vi "Methods_Insert Dividers.vi"(11 "Methods[] In":T1(array[cluster])) -> (3 "Methods[] Out":T1(array[cluster]))   [LabVIEW 2023] (continued)
"Short name (localized)"="ClearSpecCompObjCache", "Long name (localized)"="Clear Specific Compiled Object Cache"}, "Method Flags"={"IsDeprecated"=FALSE, "IsPrivate"=TRUE, "IsScripting"=FALSE, "IsNotInRun-Time"=TRUE}, "Divider"=FALSE}, {"Class Info"={"Unique ID string"="1", "Parent ID string"="", "Class Name (unlocalized)"="Application", "Class Name (localized)"="Application"}, "Method Info"={"Unique ID string"="969", "Data name"="Restart", "Short name (localized)"="Restart", "Long name (localized)"="Restart"}, "Method Flags"={"IsDeprecated"=FALSE, "IsPrivate"=FALSE, "IsScripting"=FALSE, "IsNotInRun-Time"=FALSE}, "Divider"=FALSE}, {"Class Info"={"Unique ID string"="1", "Parent ID string"="", "Class Name (unlocalized)"="Application", "Class Name (localized)"="Application"}, "Method Info"={"Unique ID string"="970", "Data name"="Get Compiled Object File", "Short name (localized)"="Get Compiled Object File", "Long name (localized)"="GetCompiledObjectFile"}, "Method Flags"={"IsDeprecated"=FALSE, "IsPrivate"=TRUE, "IsScripting"=FALSE, "IsNotInRun-Time"=FALSE}, "Divider"=FALSE}, {"Class Info"={"Unique ID string"="1", "Parent ID string"="", "Class Name (unlocalized)"="Application", "Class Name (localized)"="Application"}, "Method Info"={"Unique ID string"="971", "Data name"="ClearAppBuilderCache", "Short name (localized)"="ClearAppBuilderCache", "Long name (localized)"="Clear Application Builder Cache"}, "Method Flags"={"IsDeprecated"=FALSE, "IsPrivate"=FALSE, "IsScripting"=FALSE, "IsNotInRun-Time"=TRUE}, "Divider"=FALSE}, {"Class Info"={"Unique ID string"="1", "Parent ID string"="", "Class Name (unlocalized)"="Application", "Class Name (localized)"="Application"}, "Method Info"={"Unique ID string"="972", "Data name"="TracingTimerEnable", "Short name (localized)"="TracingTimerEnable", "Long name (localized)"="Tracing Timer Enable"}, "Method Flags"={"IsDeprecated"=FALSE, "IsPrivate"=TRUE, "IsScripting"=FALSE, "IsNotInRun-Time"=TRUE}, "Divider"=FALSE}, {"Class Info"={"Unique ID string"="1", "Parent ID string"="", "Class Name (unlocalized)"="Application", "Class Name (localized)"="Application"}, "Method Info"={"Unique ID string"="973", "Data name"="TracingTimerHarvestLogAndReset", "Short name (localized)"="TracingTimerHarvestLogAndReset", "Long name (localized)"="Tracing Timer Harvest Log And Reset"}, "Method Flags"={"IsDeprecated"=FALSE, "IsPrivate"=TRUE, "IsScripting"=FALSE, "IsNotInRun-Time"=TRUE}, "Divider"=FALSE}, {"Class Info"={"Unique ID string"="1", "Parent ID string"="", "Class Name (unlocalized)"="Application", "Class Name (localized)"="Application"}, "Method Info"={"Unique ID string"="974", "Data name"="Context.CrossContextLoadVI", "Short name (localized)"="Context.CrossContextLoadVI", "Long name (localized)"="Context:Cross Context Load Unsaved VI"}, "Method Flags"={"IsDeprecated"=FALSE, "IsPrivate"=TRUE, "IsScripting"=FALSE, "IsNotInRun-Time"=FALSE}, "Divider"=FALSE}, {"Class Info"={"Unique ID string"="1", "Parent ID string"="", "Class Name (unlocalized)"="Application", "Class Name (localized)"="Application"}, "Method Info"={"Unique ID string"="978", "Data name"="Freeze Polys", "Short name (localized)"="Freeze Polys", "Long name (localized)"="Freeze Poly VIs"}, "Method Flags"={"IsDeprecated"=FALSE, "IsPrivate"=TRUE, "IsScripting"=FALSE, "IsNotInRun-Time"=TRUE}, "Divider"=FALSE}, {"Class Info"={"Unique ID string"="1", "Parent ID string"="", "Class Name (unlocalized)"="Application", "Class Name (localized)"="Application"}, "Method Info"={"Unique ID string"="979", "Data name"="GetInstantiationVIPath", "Short name (localized)"="GetInstantiationVIPath", "Long name (localized)"="Get Instantiation VI Path"}, "Method Flags"={"IsDeprecated"=FALSE, "IsPrivate"=TRUE, "IsScripting"=FALSE, "IsNotInRun-Time"=FALSE}, "Divider"=FALSE}, {"Class Info"={"Unique ID string"="1", "Parent ID string"="", "Class Name (unlocalized)"="Application", "Class Name (localized)"="Application"}, "Method Info"={"Unique ID string"="97a", "Data name"="Change Popup Paths", "Short name (localized)"="Change Popup Paths", "Long name (localized)"="Change Control Popup RTM Paths"}, "Method Flags"={"IsDeprecated"=FALSE, "IsPrivate"=TRUE, "IsScripting"=FALSE, "IsNotInRun-Time"=TRUE}, "Divider"=FALSE}, {"Class Info"={"Unique ID string"="1", "Parent ID string"="", "Class Name (unlocalized)"="Application", "Class Name (localized)"="Application"}, "Method Info"={"Unique ID string"="97b", "Data name"="Project.NewWithPrompts", "Short name (localized)"="Project.NewWithPrompts", "Long name (localized)"="Project:New with Prompts"}, "Method Flags"={"IsDeprecated"=FALSE, "IsPrivate"=FALSE, "IsScripting"=TRUE, "IsNotInRun-Time"=TRUE}, "Divider"=FALSE}, {"Class Info"={"Unique ID string"="1", "Parent ID string"="", "Class Name (unlocalized)"="Application", "Class Name (localized)"="Application"}, "Method Info"={"Unique ID string"="97c", "Data name"="ResetCrossCompileCount", "Short name (localized)"="ResetCrossCompileCount", "Long name (localized)"="Reset Cross Compile Count"}, "Method Flags"={"IsDeprecated"=FALSE, "IsPrivate"=TRUE, "IsScripting"=FALSE, "IsNotInRun-Time"=TRUE}, "Divider"=FALSE}, {"Class Info"={"Unique ID string"="1", "Parent ID string"="", "Class Name (unlocalized)"="Application", "Class Name (localized)"="Application"}, "Method Info"={"Unique ID string"="97d", "Data name"="Get Broken VI List", "Short name (localized)"="Get Broken VI List", "Long name (localized)"="Get Broken VI List"}, "Method Flags"={"IsDeprecated"=FALSE, "IsPrivate"=TRUE, "IsScripting"=TRUE, "IsNotInRun-Time"=TRUE}, "Divider"=FALSE}, {"Class Info"={"Unique ID string"="1", "Parent ID string"="", "Class Name (unlocalized)"="Application", "Class Name (localized)"="Application"}, "Method Info"={"Unique ID string"="97e", "Data name"="Get VI.Is Global", "Short name (localized)"="Get VI.Is Global", "Long name (localized)"="Get VI:Is Global"}, "Method Flags"={"IsDeprecated"=FALSE, "IsPrivate"=TRUE, "IsScripting"=FALSE, "IsNotInRun-Time"=TRUE}, "Divider"=FALSE}, {"Class Info"={"Unique ID string"="1", "Parent ID string"="", "Class Name (unlocalized)"="Application", "Class Name (localized)"="Application"}, "Method Info"={"Unique ID string"="97f", "Data name"="Get VI.CompiledForCurrent", "Short name (localized)"="Get VI.CompiledForCurrent", "Long name (localized)"="Get VI:Compiled For Current"}, "Method Flags"={"IsDeprecated"=FALSE, "IsPrivate"=TRUE, "IsScripting"=FALSE, "IsNotInRun-Time"=TRUE}, "Divider"=FALSE}, {"Class Info"={"Unique ID string"="1", "Parent ID string"="", "Class Name (unlocalized)"="Application", "Class Name (localized)"="Application"}, "Method Info"={"Unique ID string"="980", "Data name"="LoadMSCompilerComponent", "Short name (localized)"="LoadMSCompilerComponent", "Long name (localized)"="MathScript:Load MathScript Compiler Component"}, "Method Flags"={"IsDeprecated"=FALSE, "IsPrivate"=TRUE, "IsScripting"=FALSE, "IsNotInRun-Time"=TRUE}, "Divider"=FALSE}, {"Class Info"={"Unique ID string"="1", "Parent ID string"="", "Class Name (unlocalized)"="Application", "Class Name (localized)"="Application"}, "Method Info"={"Unique ID string"="981", "Data name"="Refresh Menus", "Short name (localized)"="Refresh Menus", "Long name (localized)"="Menus:Refresh"}, "Method Flags"={"IsDeprecated"=FALSE, "IsPrivate"=FALSE, "IsScripting"=FALSE, "IsNotInRun-Time"=TRUE}, "Divider"=FALSE}, {"Class Info"={"Unique ID string"="1", "Parent ID string"="", "Class Name (unlocalized)"="Application", "Class Name (localized)"="Application"}, "Method Info"={"Unique ID string"="982", "Data name"="Library.Has Shared Variables", "Short name (localized)"="Library.Has Shared Variables", "Long name (localized)"="Library:Has Shared Variables"}, "Method Flags"={"IsDeprecated"=FALSE, "IsPrivate"=TRUE, "IsScripting"=FALSE, "IsNotInRun-Time"=TRUE}, "Divider"=FALSE}, {"Class Info"={"Unique ID string"="1", "Parent ID string"="", "Class Name (unlocalized)"="Application", "Class Name (localized)"="Application"}, "Method Info"={"Unique ID string"="983", "Data name"="UI.Cmp VIs XML", "Short name (localized)"="UI.Cmp VIs XML", "Long name (localized)"="User Interaction:Compare VIs XML"}, "Method Flags"={"IsDeprecated"=FALSE, "IsPrivate"=TRUE, "IsScripting"=FALSE, "IsNotInRun-Time"=TRUE}, "Divider"=FALSE}, {"Class Info"={"Unique ID string"="1", "Parent ID string"="", "Class Name (unlocalized)"="Application", "Class Name (localized)"="Application"}, "Method Info"={"Unique ID string"="985", "Data name"="Object Manager:Get Managers", "Short name (localized)"="Object Manager:Get Managers", "Long name (localized)"="Object Manager:Get Managers"}, "Method Flags"={"IsDeprecated"=FALSE, "IsPrivate"=TRUE, "IsScripting"=FALSE, "IsNotInRun-Time"=FALSE}, "Divider"=FALSE}, {"Class Info"={"Unique ID string"="1", "Parent ID string"="", "Class Name (unlocalized)"="Application", "Class Name (localized)"="Application"}, "Method Info"={"Unique ID string"="986", "Data name"="Object Manager:Get Classes", "Short name (localized)"="Object Manager:Get Classes", "Long name (localized)"="Object Manager:Get Classes"}, "Method Flags"={"IsDeprecated"=FALSE, "IsPrivate"=TRUE, "IsScripting"=FALSE, "IsNotInRun-Time"=FALSE}, "Divider"=FALSE}, {"Class Info"={"Unique ID string"="1", "Parent ID string"="", "Class Name (unlocalized)"="Application", "Class Name (localized)"="Application"}, "Method Info"={"Unique ID string"="987", "Data name"="Object Manager:Get Properties", "Short name (localized)"="Object Manager:Get Properties", "Long name (localized)"="Object Manager:Get Properties"}, "Method Flags"={"IsDeprecated"=FALSE, "IsPrivate"=TRUE, "IsScripting"=FALSE, "IsNotInRun-Time"=FALSE}, "Divider"=FALSE}, {"Class Info"={"Unique ID string"="1", "Parent ID string"="", "Class Name (unlocalized)"="Application", "Class Name (localized)"="Application"}, "Method Info"={"Unique ID string"="988", "Data name"="Object Manager:Show Help", "Short name (localized)"="Object Manager:Show Help", "Long name (localized)"="Object Manager:Show Help"}, "Method Flags"={"IsDeprecated"=FALSE, "IsPrivate"=TRUE, "IsScripting"=FALSE, "IsNotInRun-Time"=FALSE}, "Divider"=FALSE}, {"Class Info"={"Unique ID string"="1", "Parent ID string"="", "Class Name (unlocalized)"="Application", "Class Name (localized)"="Application"}, "Method Info"={"Unique ID string"="989", "Data name"="Get VI.Bookmarks", "Short name (localized)"="Get VI.Bookmarks", "Long name (localized)"="Get VI:Bookmarks"}, "Method Flags"={"IsDeprecated"=FALSE, "IsPrivate"=FALSE, "IsScripting"=FALSE, "IsNotInRun-Time"=FALSE}, "Divider"=FALSE}, {"Class Info"={"Unique ID string"="1", "Parent ID string"="", "Class Name (unlocalized)"="Application", "Class Name (localized)"="Application"}, "Method Info"={"Unique ID string"="98a", "Data name"="DoPostInstallObjCacheCheck", "Short name (localized)"="DoPostInstallObjCacheCheck", "Long name (localized)"="Do Post Install ObjCache Check"}, "Method Flags"={"IsDeprecated"=FALSE, "IsPrivate"=TRUE, "IsScripting"=FALSE, "IsNotInRun-Time"=TRUE}, "Divider"=FALSE}, {"Class Info"={"Unique ID string"="1", "Parent ID string"="", "Class Name (unlocalized)"="Application", "Class Name (localized)"="Application"}, "Method Info"={"Unique ID string"="98b", "Data name"="All Methods Of LVClass", "Short name (localized)"="All Methods Of LVClass", "Long name (localized)"="LabVIEW Class:All Methods of LVClass"}, "Method Flags"={"IsDeprecated"=FALSE, "IsPrivate"=FALSE, "IsScripting"=FALSE, "IsNotInRun-Time"=FALSE}, "Divider"=FALSE}, {"Class Info"={"Unique ID string"="1", "Parent ID string"="", "Class Name (unlocalized)"="Application", "Class Name (localized)"="Application"}, "Method Info"={"Unique ID string"="98c", "Data name"="LVClass Implementing VI Path", "Short name (localized)"="LVClass Implementing VI Path", "Long name (localized)"="LabVIEW Class:Get Implementing VI Path"}, "Method Flags"={"IsDeprecated"=FALSE, "IsPrivate"=FALSE, "IsScripting"=FALSE, "IsNotInRun-Time"=FALSE}, "Divider"=FALSE}, {"Class Info"={"Unique ID string"="1", "Parent ID string"="", "Class Name (unlocalized)"="Application", "Class Name (localized)"="Application"}, "Method Info"={"Unique ID string"="98d", "Data name"="Get VI.GetPrimDeps", "Short name (localized)"="Get VI.GetPrimDeps", "Long name (localized)"="Get VI:Get Prim Dependency Flags"}, "Method Flags"={"IsDeprecated"=FALSE, "IsPrivate"=TRUE, "IsScripting"=TRUE, "IsNotInRun-Time"=TRUE}, "Divider"=FALSE}, {"Class Info"={"Unique ID string"="1", "Parent ID string"="", "Class Name (unlocalized)"="Application", "Class Name (localized)"="Application"}, "Method Info"={"Unique ID string"="98e", "Data name"="IsCalleeInlined", "Short name (localized)"="IsCalleeInlined", "Long name (localized)"="Compiler:Is Callee Inlined"}, "Method Flags"={"IsDeprecated"=FALSE, "IsPrivate"=TRUE, "IsScripting"=FALSE, "IsNotInRun-Time"=FALSE}, "Divider"=FALSE}, {"Class Info"={"Unique ID string"="1", "Parent ID string"="", "Class Name (unlocalized)"="Application", "Class Name (localized)"="Application"}, "Method Info"={"Unique ID string"="98f", "Data name"="UI.ShowPaletteObjContextHelp", "Short name (localized)"="UI.ShowPaletteObjContextHelp", "Long name (localized)"="User Interaction:Show Palette Object Context Help"}, "Method Flags"={"IsDeprecated"=FALSE, "IsPrivate"=FALSE, "IsScripting"=TRUE, "IsNotInRun-Time"=TRUE}, "Divider"=FALSE}, {"Class Info"={"Unique ID string"="1", "Parent ID string"="", "Class Name (unlocalized)"="Application", "Class Name (localized)"="Application"}, "Method Info"={"Unique ID string"="990", "Data name"="Get VI.Help Info", "Short name (localized)"="Get VI.Help Info", "Long name (localized)"="Get VI:Help Info"}, "Method Flags"={"IsDeprecated"=FALSE, "IsPrivate"=FALSE, "IsScripting"=FALSE, "IsNotInRun-Time"=FALSE}, "Divider"=FALSE}, {"Class Info"={"Unique ID string"="1", "Parent ID string"="", "Class Name (unlocalized)"="Application", "Class Name (localized)"="Application"}, "Method Info"={"Unique ID string"="991", "Data name"="DSObserverCmd", "Short name (localized)"="DSObserverCmd", "Long name (localized)"="Memory Profiling:DSObserver Command"}, "Method Flags"={"IsDeprecated"=FALSE, "IsPrivate"=TRUE, "IsScripting"=FALSE, "IsNotInRun-Time"=FALSE}, "Divider"=FALSE}, {"Class Info"={"Unique ID string"="1", "Parent ID string"="", "Class Name (unlocalized)"="Application", "Class Name (localized)"="Application"}, "Method Info"={"Unique ID string"="992", "Data name"="OpenBinaryLibrary", "Short name (localized)"="OpenBinaryLibrary", "Long name (localized)"="OpenBinaryLibrary"}, "Method Flags"={"IsDeprecated"=FALSE, "IsPrivate"=TRUE, "IsScripting"=FALSE, "IsNotInRun-Time"=FALSE}, "Divider"=FALSE}, {"Class Info"={"Unique ID string"="1", "Parent ID string"="", "Class Name (unlocalized)"="Application", "Class Name (localized)"="Application"}, "Method Info"={"Unique ID string"="993", "Data name"="CloseLEIFBuildData", "Short name (localized)"="CloseLEIFBuildData", "Long name (localized)"="Close LEIF Build Data Cookie"}, "Method Flags"={"IsDeprecated"=FALSE, "IsPrivate"=TRUE, "IsScripting"=FALSE, "IsNotInRun-Time"=TRUE}, "Divider"=FALSE}, {"Class Info"={"Unique ID string"="1", "Parent ID string"="", "Class Name (unlocalized)"="Application", "Class Name (localized)"="Application"}, "Method Info"={"Unique ID string"="994", "Data name"="Build.BCRTEEnabledPackedLibrary", "Short name (localized)"="Build.BCRTEEnabledPackedLibrary", "Long name (localized)"="Build:BCRTEEnabledPackedLibrary"}, "Method Flags"={"IsDeprecated"=FALSE, "IsPrivate"=TRUE, "IsScripting"=FALSE, "IsNotInRun-Time"=TRUE}, "Divider"=FALSE}, {"Class Info"={"Unique ID string"="1", "Parent ID string"="", "Class Name (unlocalized)"="Application", "Class Name (localized)"="Application"}, "Method Info"={"Unique ID string"="995", "Data name"="PackedLibrary.IsLoadableInBinaryCompatibleLV", "Short name (localized)"="PackedLibrary.IsLoadableInBinaryCompatibleLV", "Long name (localized)"="Packed Library:Is Packed Library Loadable In Binary Compatible LabVIEW"}, "Method Flags"={"IsDeprecated"=FALSE, "IsPrivate"=TRUE, "IsScripting"=FALSE, "IsNotInRun-Time"=FALSE}, "Divider"=FALSE}, {"Class Info"={"Unique ID string"="1", "Parent ID string"="", "Class Name (unlocalized)"="Application", "Class Name (localized)"="Application"}, "Method Info"={"Unique ID string"="996", "Data name"="SetGlobalBackwardCompatibleLoadEnabled", "Short name (localized)"="SetGlobalBackwardCompatibleLoadEnabled", "Long name (localized)"="BCRTE:SetGlobalBackwardCompatibleLoadEnabled"}, "Method Flags"={"IsDeprecated"=FALSE, "IsPrivate"=TRUE, "IsScripting"=FALSE, "IsNotInRun-Time"=FALSE}, "Divider"=FALSE}, {"Class Info"={"Unique ID string"="1", "Parent ID string"="", "Class Name (unlocalized)"="Application", "Class Name (localized)"="Application"}, "Method Info"={"Unique ID string"="997", "Data name"="IsGlobalBackwardCompatibleLoadEnabled", "Short name (localized)"="IsGlobalBackwardCompatibleLoadEnabled", "Long name (localized)"="BCRTE:IsGlobalBackwardCompatibleLoadEnabled"}, "Method Flags"={"IsDeprecated"=FALSE, "IsPrivate"=TRUE, "IsScripting"=FALSE, "IsNotInRun-Time"=FALSE}, "Divider"=FALSE}, {"Class Info"={"Unique ID string"="1", "Parent ID string"="", "Class Name (unlocalized)"="Application", "Class Name (localized)"="Application"}, "Method Info"={"Unique ID string"="998", "Data name"="Linker.Read Info From File Exclude LVRT Shipped Libs", "Short name (localized)"="Linker.Read Info From File Exclude LVRT Shipped Libs", "Long name (localized)"="Linker:Read Info From File Exclude LVRT Shipped Libs"}, "Method Flags"={"IsDeprecated"=FALSE, "IsPrivate"=TRUE, "IsScripting"=FALSE, "IsNotInRun-Time"=TRUE}, "Divider"=FALSE}, {"Class Info"={"Unique ID string"="1", "Parent ID string"="", "Class Name (unlocalized)"="Application", "Class Name (localized)"="Application"}, "Method Info"={"Unique ID string"="999", "Data name"="Project.Open And Suppress Source-Only", "Short name (localized)"="Project.Open And Suppress Source-Only", "Long name (localized)"="Project:Open And Suppress Source-Only"}, "Method Flags"={"IsDeprecated"=FALSE, "IsPrivate"=FALSE, "IsScripting"=TRUE, "IsNotInRun-Time"=TRUE}, "Divider"=FALSE}, {"Class Info"={"Unique ID string"="1", "Parent ID string"="", "Class Name (unlocalized)"="Application", "Class Name (localized)"="Application"}, "Method Info"={"Unique ID string"="99a", "Data name"="NativeEventTracingSetup", "Short name (localized)"="NativeEventTracingSetup", "Long name (localized)"="NativeEventTracing:Setup"}, "Method Flags"={"IsDeprecated"=FALSE, "IsPrivate"=TRUE, "IsScripting"=FALSE, "IsNotInRun-Time"=FALSE}, "Divider"=FALSE}, {"Class Info"={"Unique ID string"="1", "Parent ID string"="", "Class Name (unlocalized)"="Application", "Class Name (localized)"="Application"}, "Method Info"={"Unique ID string"="99b", "Data name"="Get VI.ConPane CRC v3", "Short name (localized)"="Get VI.ConPane CRC v3", "Long name (localized)"="Get VI:ConPane CRC v3"}, "Method Flags"={"IsDeprecated"=FALSE, "IsPrivate"=TRUE, "IsScripting"=FALSE, "IsNotInRun-Time"=FALSE}, "Divider"=FALSE}, {"Class Info"={"Unique ID string"="1", "Parent ID string"="", "Class Name (unlocalized)"="Application", "Class Name (localized)"="Application"}, "Method Info"={"Unique ID string"="99c", "Data name"="Get VI.ConPane CRC Ignore DD v2", "Short name (localized)"="Get VI.ConPane CRC Ignore DD v2", "Long name (localized)"="Get VI:ConPane CRC Ignore Dynamic Dispatch v2"}, "Method Flags"={"IsDeprecated"=FALSE, "IsPrivate"=TRUE, "IsScripting"=FALSE, "IsNotInRun-Time"=FALSE}, "Divider"=FALSE}, {"Class Info"={"Unique ID string"="2", "Parent ID string"="", "Class Name (unlocalized)"="VI", "Class Name (localized)"="VI"}, "Method Info"={"Unique ID string"="3e8", "Data name"="VI Strings.Export", "Short name (localized)"="VI Strings.Export", "Long name (localized)"="VI Strings:Export"}, "Method Flags"={"IsDeprecated"=FALSE, "IsPrivate"=FALSE, "IsScripting"=FALSE, "IsNotInRun-Time"=TRUE}, "Divider"=FALSE}, {"Class Info"={"Unique ID string"="2", "Parent ID string"="", "Class Name (unlocalized)"="VI", "Class Name (localized)"="VI"}, "Method Info"={"Unique ID string"="3e9", "Data name"="VI Strings.Import", "Short name (localized)"="VI Strings.Import", "Long name (localized)"="VI Strings:Import"}, "Method Flags"={"IsDeprecated"=FALSE, "IsPrivate"=FALSE, "IsScripting"=FALSE, "IsNotInRun-Time"=FALSE}, "Divider"=FALSE}, {"Class Info"={"Unique ID string"="2", "Parent ID string"="", "Class Name (unlocalized)"="VI", "Class Name (localized)"="VI"}, "Method Info"={"Unique ID string"="3ea", "Data name"="Save.Instrument", "Short name (localized)"="Save.Instrument", "Long name (localized)"="Save:Instrument"}, "Method Flags"={"IsDeprecated"=FALSE, "IsPrivate"=FALSE, "IsScripting"=FALSE, "IsNotInRun-Time"=TRUE}, "Divider"=FALSE}, {"Class Info"={"Unique ID string"="2", "Parent ID string"="", "Class Name (unlocalized)"="VI", "Class Name (localized)"="VI"}, "Method Info"={"Unique ID string"="3eb", "Data name"="Run VI", "Short name (localized)"="Run VI", "Long name (localized)"="Run VI"}, "Method Flags"={"IsDeprecated"=FALSE, "IsPrivate"=FALSE, "IsScripting"=FALSE, "IsNotInRun-Time"=FALSE}, "Divider"=FALSE}, {"Class Info"={"Unique ID string"="2", "Parent ID string"="", "Class Name (unlocalized)"="VI", "Class Name (localized)"="VI"}, "Method Info"={"Unique ID string"="3ec", "Data name"="Abort VI", "Short name (localized)"="Abort VI", "Long name (localized)"="Abort VI"}, "Method Flags"={"IsDeprecated"=FALSE, "IsPrivate"=FALSE, "IsScripting"=FALSE, "IsNotInRun-Time"=FALSE}, "Divider"=FALSE}, {"Class Info"={"Unique ID string"="2", "Parent ID string"="", "Class Name (unlocalized)"="VI", "Class Name (localized)"="VI"}, "Method Info"={"Unique ID string"="3ed", "Data name"="Print.VI To Printer", "Short name (localized)"="Print.VI To Printer", "Long name (localized)"="Print:VI To Printer"}, "Method Flags"={"IsDeprecated"=FALSE, "IsPrivate"=FALSE, "IsScripting"=FALSE, "IsNotInRun-Time"=FALSE}, "Divider"=FALSE}, {"Class Info"={"Unique ID string"="2", "Parent ID string"="", "Class Name (unlocalized)"="VI", "Class Name (localized)"="VI"}, "Method Info"={"Unique ID string"="3ee", "Data name"="Print.VI To HTML", "Short name (localized)"="Print.VI To HTML", "Long name (localized)"="Print:VI To HTML"}, "Method Flags"={"IsDeprecated"=FALSE, "IsPrivate"=FALSE, "IsScripting"=FALSE, "IsNotInRun-Time"=TRUE}, "Divider"=FALSE}, {"Class Info"={"Unique ID string"="2", "Parent ID string"="", "Class Name (unlocalized)"="VI", "Class Name (localized)"="VI"}, "Method Info"={"Unique ID string"="3ef", "Data name"="Print.VI To RTF", "Short name (localized)"="Print.VI To RTF", "Long name (localized)"="Print:VI To RTF"}, "Method Flags"={"IsDeprecated"=FALSE, "IsPrivate"=FALSE, "IsScripting"=FALSE, "IsNotInRun-Time"=TRUE}, "Divider"=FALSE}, {"Class Info"={"Unique ID string"="2", "Parent ID string"="", "Class Name (unlocalized)"="VI", "Class Name (localized)"="VI"}, "Method Info"={"Unique ID string"="3f0", "Data name"="Print.VI To Text", "Short name (localized)"="Print.VI To Text", "Long name (localized)"="Print:VI To Text"}, "Method Flags"={"IsDeprecated"=FALSE, "IsPrivate"=FALSE, "IsScripting"=FALSE, "IsNotInRun-Time"=TRUE}, "Divider"=FALSE}, {"Class Info"={"Unique ID string"="2", "Parent ID string"="", "Class Name (unlocalized)"="VI", "Class Name (localized)"="VI"}, "Method Info"={"Unique ID string"="3f3", "Data name"="Default Vals.Make Curr Default", "Short name (localized)"="Default Vals.Make Curr Default", "Long name (localized)"="Default Values:Make Current Default"}, "Method Flags"={"IsDeprecated"=FALSE, "IsPrivate"=FALSE, "IsScripting"=FALSE, "IsNotInRun-Time"=TRUE}, "Divider"=FALSE}, {"Class Info"={"Unique ID string"="2", "Parent ID string"="", "Class Name (unlocalized)"="VI", "Class Name (localized)"="VI"}, "Method Info"={"Unique ID string"="3f4", "Data name"="Default Vals.Reinit All", "Short name (localized)"="Default Vals.Reinit All", "Long name (localized)"="Default Values:Reinitialize All To Default"}, "Method Flags"={"IsDeprecated"=FALSE, "IsPrivate"=FALSE, "IsScripting"=FALSE, "IsNotInRun-Time"=FALSE}, "Divider"=FALSE}, {"Class Info"={"Unique ID string"="2", "Parent ID string"="", "Class Name (unlocalized)"="VI", "Class Name (localized)"="VI"}, "Method Info"={"Unique ID string"="3fa", "Data name"="Revert VI", "Short name (localized)"="Revert VI", "Long name (localized)"="Revert VI"}, "Method Flags"={"IsDeprecated"=FALSE, "IsPrivate"=FALSE, "IsScripting"=FALSE, "IsNotInRun-Time"=TRUE}, "Divider"=FALSE}, {"Class Info"={"Unique ID string"="2", "Parent ID string"="", "Class Name (unlocalized)"="VI", "Class Name (localized)"="VI"}, "Method Info"={"Unique ID string"="3fb", "Data name"="Print.Panel To Printer", "Short name (localized)"="Print.Panel To Printer", "Long name (localized)"="Print:Panel To Printer"}, "Method Flags"={"IsDeprecated"=FALSE, "IsPrivate"=FALSE, "IsScripting"=FALSE, "IsNotInRun-Time"=FALSE}, "Divider"=FALSE}, {"Class Info"={"Unique ID string"="2", "Parent ID string"="", "Class Name (unlocalized)"="VI", "Class Name (localized)"="VI"}, "Method Info"={"Unique ID string"="3fd", "Data name"="Lock State.Get", "Short name (localized)"="Lock State.Get", "Long name (localized)"="Lock State:Get"}, "Method Flags"={"IsDeprecated"=FALSE, "IsPrivate"=FALSE, "IsScripting"=FALSE, "IsNotInRun-Time"=FALSE}, "Divider"=FALSE}, {"Class Info"={"Unique ID string"="2", "Parent ID string"="", "Class Name (unlocalized)"="VI", "Class Name (localized)"="VI"}, "Method Info"={"Unique ID string"="3fe", "Data name"="Lock State.Set", "Short name (localized)"="Lock State.Set", "Long name (localized)"="Lock State:Set"}, "Method Flags"={"IsDeprecated"=FALSE, "IsPrivate"=FALSE, "IsScripting"=FALSE, "IsNotInRun-Time"=TRUE}, "Divider"=FALSE}, {"Class Info"={"Unique ID string"="2", "Parent ID string"="", "Class Name (unlocalized)"="VI", "Class Name (localized)"="VI"}, "Method Info"={"Unique ID string"="3ff", "Data name"="Private Save Instrument", "Short name (localized)"="Private Save Instrument", "Long name (localized)"="Save:Instrument (Private)"}, "Method Flags"={"IsDeprecated"=FALSE, "IsPrivate"=TRUE, "IsScripting"=FALSE, "IsNotInRun-Time"=TRUE}, "Divider"=FALSE}, {"Class Info"={"Unique ID string"="2", "Parent ID string"="", "Class Name (unlocalized)"="VI", "Class Name (localized)"="VI"}, "Method Info"={"Unique ID string"="400", "Data name"="Save.For Previous", "Short name (localized)"="Save.For Previous", "Long name (localized)"="Save:For Previous"}, "Method Flags"={"IsDeprecated"=FALSE, "IsPrivate"=FALSE, "IsScripting"=FALSE, "IsNotInRun-Time"=TRUE}, "Divider"=FALSE}, {"Class Info"={"Unique ID string"="2", "Parent ID string"="", "Class Name (unlocalized)"="VI", "Class Name (localized)"="VI"}, "Method Info"={"Unique ID string"="401", "Data name"="Empty", "Short name (localized)"="Empty", "Long name (localized)"="Empty"}, "Method Flags"={"IsDeprecated"=FALSE, "IsPrivate"=FALSE, "IsScripting"=TRUE, "IsNotInRun-Time"=TRUE}, "Divider"=FALSE}, {"Class Info"={"Unique ID string"="2", "Parent ID string"="", "Class Name (unlocalized)"="VI", "Class Name (localized)"="VI"}, "Method Info"={"Unique ID string"="402", "Data name"="Transaction.Begin Undo", "Short name (localized)"="Transaction.Begin Undo", "Long name (localized)"="Transaction:Begin Undo"}, "Method Flags"={"IsDeprecated"=FALSE, "IsPrivate"=FALSE, "IsScripting"=TRUE, "IsNotInRun-Time"=TRUE}, "Divider"=FALSE}, {"Class Info"={"Unique ID string"="2", "Parent ID string"="", "Class Name (unlocalized)"="VI", "Class Name (localized)"="VI"}, "Method Info"={"Unique ID string"="403", "Data name"="Transaction.End Undo", "Short name (localized)"="Transaction.End Undo", "Long name (localized)"="Transaction:End Undo"}, "Method Flags"={"IsDeprecated"=FALSE, "IsPrivate"=FALSE, "IsScripting"=TRUE, "IsNotInRun-Time"=TRUE}, "Divider"=FALSE}, {"Class Info"={"Unique ID string"="2", "Parent ID string"="", "Class Name (unlocalized)"="VI", "Class Name (localized)"="VI"}, "Method Info"={"Unique ID string"="407", "Data name"="VI Icon.Set from File", "Short name (localized)"="VI Icon.Set from File", "Long name (localized)"="VI Icon:Set From File"}, "Method Flags"={"IsDeprecated"=FALSE, "IsPrivate"=FALSE, "IsScripting"=FALSE, "IsNotInRun-Time"=TRUE}, "Divider"=FALSE}, {"Class Info"={"Unique ID string"="2", "Parent ID string"="", "Class Name (unlocalized)"="VI", "Class Name (localized)"="VI"}, "Method Info"={"Unique ID string"="409", "Data name"="Tag.Remove Tags", "Short name (localized)"="Tag.Remove Tags", "Long name (localized)"="Tag:Remove Tags"}, "Method Flags"={"IsDeprecated"=FALSE, "IsPrivate"=TRUE, "IsScripting"=FALSE, "IsNotInRun-Time"=FALSE}, "Divider"=FALSE}, {"Class Info"={"Unique ID string"="2", "Parent ID string"="", "Class Name (unlocalized)"="VI", "Class Name (localized)"="VI"}, "Method Info"={"Unique ID string"="40a", "Data name"="Tag.Set Tags", "Short name (localized)"="Tag.Set Tags", "Long name (localized)"="Tag:Set Tags"}, "Method Flags"={"IsDeprecated"=FALSE, "IsPrivate"=TRUE, "IsScripting"=FALSE, "IsNotInRun-Time"=FALSE}, "Divider"=FALSE}, {"Class Info"={"Unique ID string"="2", "Parent ID string"="", "Class Name (unlocalized)"="VI", "Class Name (localized)"="VI"}, "Method Info"={"Unique ID string"="40b", "Data name"="Tag.Set Persistence", "Short name (localized)"="Tag.Set Persistence", "Long name (localized)"="Tag:Set Persistence"}, "Method Flags"={"IsDeprecated"=FALSE, "IsPrivate"=TRUE, "IsScripting"=FALSE, "IsNotInRun-Time"=FALSE}, "Divider"=FALSE}, {"Class Info"={"Unique ID string"="2", "Parent ID string"="", "Class Name (unlocalized)"="VI", "Class Name (localized)"="VI"}, "Method Info"={"Unique ID string"="40c", "Data name"="Tag.Remove All Tags", "Short name (localized)"="Tag.Remove All Tags", "Long name (localized)"="Tag:Remove All Tags"}, "Method Flags"={"IsDeprecated"=FALSE, "IsPrivate"=TRUE, "IsScripting"=FALSE, "IsNotInRun-Time"=FALSE}, "Divider"=FALSE}, {"Class Info"={"Unique ID string"="2", "Parent ID string"="", "Class Name (unlocalized)"="VI", "Class Name (localized)"="VI"}, "Method Info"={"Unique ID string"="40d", "Data name"="Tag.Set Tag", "Short name (localized)"="Tag.Set Tag", "Long name (localized)"="Tag:Set Tag"}, "Method Flags"={"IsDeprecated"=FALSE, "IsPrivate"=TRUE, "IsScripting"=FALSE, "IsNotInRun-Time"=FALSE}, "Divider"=FALSE}, {"Class Info"={"Unique ID string"="2", "Parent ID string"="", "Class Name (unlocalized)"="VI", "Class Name (localized)"="VI"}, "Method Info"={"Unique ID string"="40e", "Data name"="Tag.Get Tag", "Short name (localized)"="Tag.Get Tag", "Long name (localized)"="Tag:Get Tag"}, "Method Flags"={"IsDeprecated"=FALSE, "IsPrivate"=TRUE, "IsScripting"=FALSE, "IsNotInRun-Time"=FALSE}, "Divider"=FALSE}, {"Class Info"={"Unique ID string"="2", "Parent ID string"="", "Class Name (unlocalized)"="VI", "Class Name (localized)"="VI"}, "Method Info"={"Unique ID string"="40f", "Data name"="Tag.Remove Tag", "Short name (localized)"="Tag.Remove Tag", "Long name (localized)"="Tag:Remove Tag"}, "Method Flags"={"IsDeprecated"=FALSE, "IsPrivate"=TRUE, "IsScripting"=FALSE, "IsNotInRun-Time"=FALSE}, "Divider"=FALSE}, {"Class Info"={"Unique ID string"="2", "Parent ID string"="", "Class Name (unlocalized)"="VI", "Class Name (localized)"="VI"}, "Method Info"={"Unique ID string"="410", "Data name"="BD.Remove Bad Wires", "Short name (localized)"="BD.Remove Bad Wires", "Long name (localized)"="Block Diagram:Remove Bad Wires"}, "Method Flags"={"IsDeprecated"=FALSE, "IsPrivate"=FALSE, "IsScripting"=TRUE, "IsNotInRun-Time"=TRUE}, "Divider"=FALSE}, {"Class Info"={"Unique ID string"="2", "Parent ID string"="", "Class Name (unlocalized)"="VI", "Class Name (localized)"="VI"}, "Method Info"={"Unique ID string"="411", "Data name"="Fake Exec State", "Short name (localized)"="Fake Exec State", "Long name (localized)"="Fake Exec State"}, "Method Flags"={"IsDeprecated"=FALSE, "IsPrivate"=TRUE, "IsScripting"=TRUE, "IsNotInRun-Time"=FALSE}, "Divider"=FALSE}, {"Class Info"={"Unique ID string"="2", "Parent ID string"="", "Class Name (unlocalized)"="VI", "Class Name (localized)"="VI"}, "Method Info"={"Unique ID string"="412", "Data name"="Generate VHDL", "Short name (localized)"="Generate VHDL", "Long name (localized)"="Generate VHDL"}, "Method Flags"={"IsDeprecated"=FALSE, "IsPrivate"=TRUE, "IsScripting"=TRUE, "IsNotInRun-Time"=TRUE}, "Divider"=FALSE}, {"Class Info"={"Unique ID string"="2", "Parent ID string"="", "Class Name (unlocalized)"="VI", "Class Name (localized)"="VI"}, "Method Info"={"Unique ID string"="413", "Data name"="Save.Run-Time Menu", "Short name (localized)"="Save.Run-Time Menu", "Long name (localized)"="Save:Run-Time Menu"}, "Method Flags"={"IsDeprecated"=FALSE, "IsPrivate"=FALSE, "IsScripting"=FALSE, "IsNotInRun-Time"=TRUE}, "Divider"=FALSE}, {"Class Info"={"Unique ID string"="2", "Parent ID string"="", "Class Name (unlocalized)"="VI", "Class Name (localized)"="VI"}, "Method Info"={"Unique ID string"="414", "Data name"="Disconnect Polys And Typedefs", "Short name (localized)"="Disconnect Polys And Typedefs", "Long name (localized)"="Disconnect Polys And Typedefs"}, "Method Flags"={"IsDeprecated"=FALSE, "IsPrivate"=TRUE, "IsScripting"=FALSE, "IsNotInRun-Time"=TRUE}, "Divider"=FALSE}, {"Class Info"={"Unique ID string"="2", "Parent ID string"="", "Class Name (unlocalized)"="VI", "Class Name (localized)"="VI"}, "Method Info"={"Unique ID string"="415", "Data name"="Print.Panel To PostScript", "Short name (localized)"="Print.Panel To PostScript", "Long name (localized)"="Print:Panel To PostScript"}, "Method Flags"={"IsDeprecated"=FALSE, "IsPrivate"=FALSE, "IsScripting"=TRUE, "IsNotInRun-Time"=FALSE}, "Divider"=FALSE}, {"Class Info"={"Unique ID string"="2", "Parent ID string"="", "Class Name (unlocalized)"="VI", "Class Name (localized)"="VI"}, "Method Info"={"Unique ID string"="418", "Data name"="VI Icon.Save to File", "Short name (localized)"="VI Icon.Save to File", "Long name (localized)"="VI Icon:Save To File"}, "Method Flags"={"IsDeprecated"=FALSE, "IsPrivate"=FALSE, "IsScripting"=FALSE, "IsNotInRun-Time"=TRUE}, "Divider"=FALSE}, {"Class Info"={"Unique ID string"="2", "Parent ID string"="", "Class Name (unlocalized)"="VI", "Class Name (localized)"="VI"}, "Method Info"={"Unique ID string"="419", "Data name"="Clear History", "Short name (localized)"="Clear History", "Long name (localized)"="Clear History"}, "Method Flags"={"IsDeprecated"=FALSE, "IsPrivate"=FALSE, "IsScripting"=FALSE, "IsNotInRun-Time"=TRUE}, "Divider"=FALSE}, {"Class Info"={"Unique ID string"="2", "Parent ID string"="", "Class Name (unlocalized)"="VI", "Class Name (localized)"="VI"}, "Method Info"={"Unique ID string"="41a", "Data name"="Save.To Buffer", "Short name (localized)"="Save.To Buffer", "Long name (localized)"="Save:To Buffer"}, "Method Flags"={"IsDeprecated"=FALSE, "IsPrivate"=TRUE, "IsScripting"=FALSE, "IsNotInRun-Time"=FALSE}, "Divider"=FALSE}, {"Class Info"={"Unique ID string"="2", "Parent ID string"="", "Class Name (unlocalized)"="VI", "Class Name (localized)"="VI"}, "Method Info"={"Unique ID string"="41b", "Data name"="Ctrl Val.Set", "Short name (localized)"="Ctrl Val.Set", "Long name (localized)"="Control Value:Set"}, "Method Flags"={"IsDeprecated"=FALSE, "IsPrivate"=FALSE, "IsScripting"=FALSE, "IsNotInRun-Time"=FALSE}, "Divider"=FALSE}, {"Class Info"={"Unique ID string"="2", "Parent ID string"="", "Class Name (unlocalized)"="VI", "Class Name (localized)"="VI"}, "Method Info"={"Unique ID string"="41c", "Data name"="Ctrl Val.Get", "Short name (localized)"="Ctrl Val.Get", "Long name (localized)"="Control Value:Get"}, "Method Flags"={"IsDeprecated"=FALSE, "IsPrivate"=FALSE, "IsScripting"=FALSE, "IsNotInRun-Time"=FALSE}, "Divider"=FALSE}, {"Class Info"={"Unique ID string"="2", "Parent ID string"="", "Class Name (unlocalized)"="VI", "Class Name (localized)"="VI"}, "Method Info"={"Unique ID string"="41d", "Data name"="Ctrl Val.Get All", "Short name (localized)"="Ctrl Val.Get All", "Long name (localized)"="Control Value:Get All"}, "Method Flags"={"IsDeprecated"=FALSE, "IsPrivate"=FALSE, "IsScripting"=FALSE, "IsNotInRun-Time"=FALSE}, "Divider"=FALSE}, {"Class Info"={"Unique ID string"="2", "Parent ID string"="", "Class Name (unlocalized)"="VI", "Class Name (localized)"="VI"}, "Method Info"={"Unique ID string"="41f", "Data name"="Save.Target Instrument", "Short name (localized)"="Save.Target Instrument", "Long name (localized)"="Save:Target Instrument"}, "Method Flags"={"IsDeprecated"=FALSE, "IsPrivate"=TRUE, "IsScripting"=FALSE, "IsNotInRun-Time"=TRUE}, "Divider"=FALSE}, {"Class Info"={"Unique ID string"="2", "Parent ID string"="", "Class Name (unlocalized)"="VI", "Class Name (localized)"="VI"}, "Method Info"={"Unique ID string"="421", "Data name"="VI Icon.Get as Image Data", "Short name (localized)"="VI Icon.Get as Image Data", "Long name (localized)"="VI Icon:Get As Image Data"}, "Method Flags"={"IsDeprecated"=FALSE, "IsPrivate"=FALSE, "IsScripting"=FALSE, "IsNotInRun-Time"=FALSE}, "Divider"=FALSE}, {"Class Info"={"Unique ID string"="2", "Parent ID string"="", "Class Name (unlocalized)"="VI", "Class Name (localized)"="VI"}, "Method Info"={"Unique ID string"="422", "Data name"="VI Icon.Set from Image Data", "Short name (localized)"="VI Icon.Set from Image Data", "Long name (localized)"="VI Icon:Set From Image Data"}, "Method Flags"={"IsDeprecated"=FALSE, "IsPrivate"=FALSE, "IsScripting"=FALSE, "IsNotInRun-Time"=TRUE}, "Divider"=FALSE}, {"Class Info"={"Unique ID string"="2", "Parent ID string"="", "Class Name (unlocalized)"="VI", "Class Name (localized)"="VI"}, "Method Info"={"Unique ID string"="423", "Data name"="FP.Get Image", "Short name (localized)"="FP.Get Image", "Long name (localized)"="Front Panel:Get Image"}, "Method Flags"={"IsDeprecated"=FALSE, "IsPrivate"=FALSE, "IsScripting"=FALSE, "IsNotInRun-Time"=FALSE}, "Divider"=FALSE}, {"Class Info"={"Unique ID string"="2", "Parent ID string"="", "Class Name (unlocalized)"="VI", "Class Name (localized)"="VI"}, "Method Info"={"Unique ID string"="425", "Data name"="FP.Close", "Short name (localized)"="FP.Close", "Long name (localized)"="Front Panel:Close"}, "Method Flags"={"IsDeprecated"=FALSE, "IsPrivate"=FALSE, "IsScripting"=FALSE, "IsNotInRun-Time"=FALSE}, "Divider"=FALSE}, {"Class Info"={"Unique ID string"="2", "Parent ID string"="", "Class Name (unlocalized)"="VI", "Class Name (localized)"="VI"}, "Method Info"={"Unique ID string"="426", "Data name"="FP.Get Image Scaled", "Short name (localized)"="FP.Get Image Scaled", "Long name (localized)"="Front Panel:Get Image Scaled"}, "Method Flags"={"IsDeprecated"=FALSE, "IsPrivate"=FALSE, "IsScripting"=FALSE, "IsNotInRun-Time"=FALSE}, "Divider"=FALSE}, {"Class Info"={"Unique ID string"="2", "Parent ID string"="", "Class Name (unlocalized)"="VI", "Class Name (localized)"="VI"}, "Method Info"={"Unique ID string"="427", "Data name"="VI Hier.Get Signature", "Short name (localized)"="VI Hier.Get Signature", "Long name (localized)"="VI Hierarchy:Get Signature"}, "Method Flags"={"IsDeprecated"=FALSE, "IsPrivate"=TRUE, "IsScripting"=FALSE, "IsNotInRun-Time"=FALSE}, "Divider"=FALSE}, {"Class Info"={"Unique ID string"="2", "Parent ID string"="", "Class Name (unlocalized)"="VI", "Class Name (localized)"="VI"}, "Method Info"={"Unique ID string"="428", "Data name"="Transaction.Undo", "Short name (localized)"="Transaction.Undo", "Long name (localized)"="Transaction:Undo"}, "Method Flags"={"IsDeprecated"=FALSE, "IsPrivate"=FALSE, "IsScripting"=TRUE, "IsNotInRun-Time"=TRUE}, "Divider"=FALSE}, {"Class Info"={"Unique ID string"="2", "Parent ID string"="", "Class Name (unlocalized)"="VI", "Class Name (localized)"="VI"}, "Method Info"={"Unique ID string"="429", "Data name"="Transaction.Redo", "Short name (localized)"="Transaction.Redo", "Long name (localized)"="Transaction:Redo"}, "Method Flags"={"IsDeprecated"=FALSE, "IsPrivate"=FALSE, "IsScripting"=TRUE, "IsNotInRun-Time"=TRUE}, "Divider"=FALSE}, {"Class Info"={"Unique ID string"="2", "Parent ID string"="", "Class Name (unlocalized)"="VI", "Class Name (localized)"="VI"}, "Method Info"={"Unique ID string"="42a", "Data name"="Transaction.Fail", 
